vi "mlink_dsp_signal_read.vi"(4 "tiemout":i32=1500, 6 "count":i32=1, 8 "error in (no error)":errorcluster, 9 "signal size":i32=1, 10 "signal ID":i32=1, 11 "connection ID":i32=-1) -> (0 "error out":errorcluster, 2 "data out":dbl[][](array[numeric]), 3 "connection ID out":i32)   [LabVIEW 2009, in "MicroDAQ.lvlib" / "mlink.lvlib"]
uses:
  <instrlib>/MicroDAQ/Mlink library wraper/mlink.lvlib
  <instrlib>/MicroDAQ/MLink32.dll
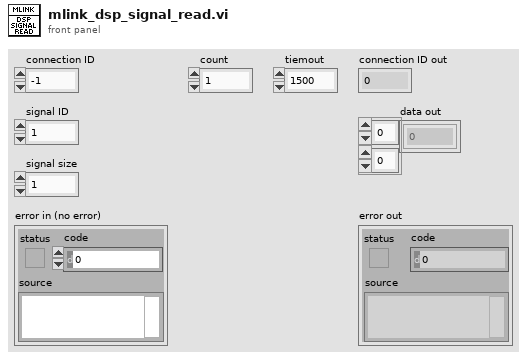
[diagram p1: front panel]
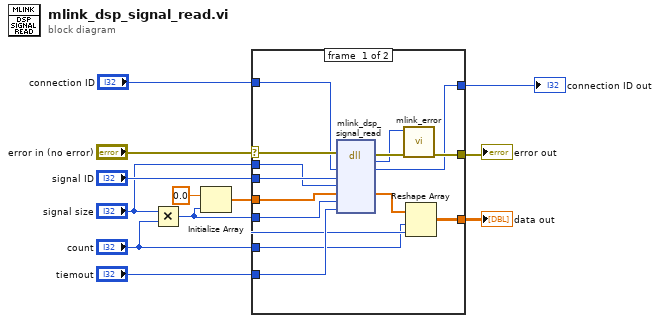
[diagram p0: block diagram]
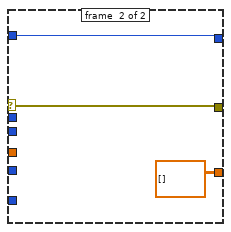
[diagram p2: hidden frame]
diagram:
  n1 = Multiply(x="signal size", y="count") -> (x*y=w4:i32)
  n2 = Initialize Array(0.0 ("element"), w4) -> (w9:dbl[])
  n3 = case shown="No Error" "error in (no error)" {
    selector: "error in (no error)" -> [w25 w29]
    tunnel: "signal ID" -> [w26 _]
    tunnel: w9 -> [w24 _]
    tunnel: [w22 dbl[][] [] ("data")] -> w8
    tunnel: "tiemout" -> [w21 _]
    tunnel: "signal size" -> [w20 _]
    tunnel: "count" -> [w19 _]
    tunnel: w4 -> [w18 _]
    tunnel: [w17 w29] -> w3
    tunnel: "connection ID" -> [w14 w27]
    tunnel: [w13 w27] -> w1
    frame #0 {
      n4 = dll-call lib="C:/Program Files (x86)/National Instruments/LabVIEW 2009/instr.lib/MicroDAQ/MLink32.dll" fn="mlink_dsp_signal_read"(error in=w25, "link_fd"=w14, "signal_id"=w26, "signal_size"=w20, "data"=w24, "data_size"=w18, "tiemout"=w21) -> (error out=w16:errorcluster, "return type"=w15:i32, "link_fd"=w13:i32, "data"=w23:dbl[])  [unwired: 6 in, 1 out]
      n5 = call <instrlib>:"mlink_error.vi"("error in (no error)"=w16, "error code"=w15) -> ("error out"=w17:errorcluster)  [unwired: 9 in]
      n6 = Reshape Array(w23, w19, w20) -> (w22:dbl[][])
    }
    frame #1 {
    }
  }
  "error out" <- w3
  "data out" <- w8
  "connection ID out" <- w1
